vi "Percent Error.vi"(10 "Expected":dbl, 11 "Observed":dbl) -> (3 "Percent Error":dbl)   [LabVIEW 2019]
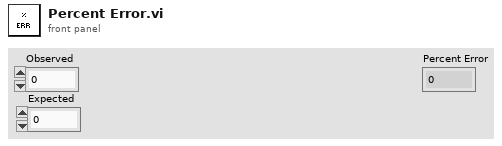
[diagram p1: front panel]
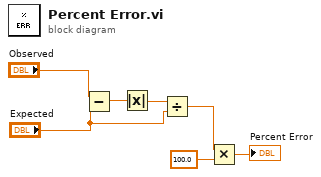
[diagram p0: block diagram]
diagram:
  n1 = Subtract(x="Observed", y="Expected") -> (x-y=w6:dbl)
  n2 = Absolute Value(x=w6) -> (abs(x)=w5:dbl)
  n3 = Divide(x=w5, y="Expected") -> (x/y=w3:dbl)
  n4 = Multiply(x=w3, y=100.0) -> (x*y=→"Percent Error":dbl)
